vi "PDC_SetLUTUserParam.vi"(6 "Params":T1, 8 "error in (no error)":errorcluster, 9 "LUTMode":u32, 10 "ChildNo":u32, 11 "DeviceNo":u32) -> (0 "error out":errorcluster, 3 "ReturnValue":u32, 4 "ErrorCode":u32)   [LabVIEW 2015]
doc: "This VI sets the pre-LUT parameter of the specified child device."
uses:
  PDCLIB.dll
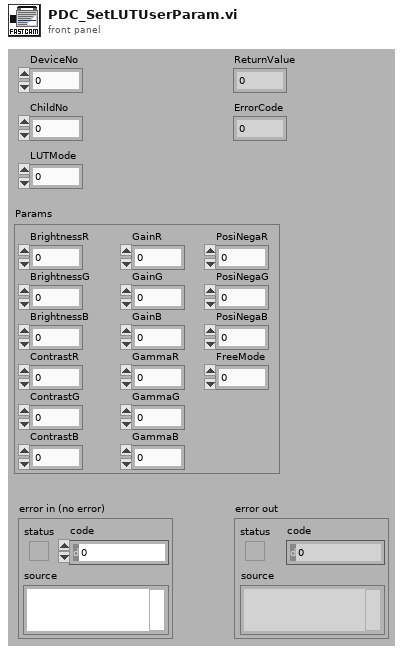
[diagram p1: front panel]
types:
  T1 = cluster{"BrightnessR":i32, "BrightnessG":i32, "BrightnessB":i32, "ContrastR":i32, "ContrastG":i32, "ContrastB":i32, "GainR":dbl, "GainG":dbl, "GainB":dbl, "GammaR":dbl, "GammaG":dbl, "GammaB":dbl, "PosiNegaR":u8, "PosiNegaG":u8, "PosiNegaB":u8, "FreeMode":u8}
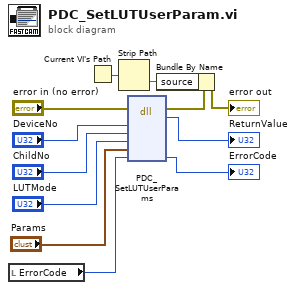
[diagram p0: block diagram]
diagram:
  n1 = local read "ErrorCode"() -> (w9:u32)
  n2 = Current VI's Path() -> (path=w3:path)
  n3 = Strip Path(path=w3) -> (name=w4:string)  [unwired: 1 out]
  n4 = dll-call lib="PDCLIB.dll" fn="PDC_SetLUTUserParams"(error in="error in (no error)", "nDeviceNo"="DeviceNo", "nChildNo"="ChildNo", "nLUTMode"="LUTMode", "pParams"="Params", "pErrorCode"=w9) -> (error out=w2:errorcluster, "return type"=→"ReturnValue":u32, "pErrorCode"=→"ErrorCode":u32)  [unwired: 6 in, 1 out]
  n5 = Bundle By Name(cluster=w2, "source"=w4) -> (→"error out":errorcluster)
